vi "ReadInnerValue.vi"(8 "error in (no error)":errorcluster, 11 "Arduino in":refnum<class "Arduino.lvclass">) -> (0 "error out":errorcluster, 3 "Arduino out":refnum<class "Arduino.lvclass">)   [LabVIEW 2013, in "Arduino.lvclass"]
uses:
  Arduino.lvclass
panel:
  out "Value":dbl
  in  "Stop_Marker":string
  in  "Start_Marker":string
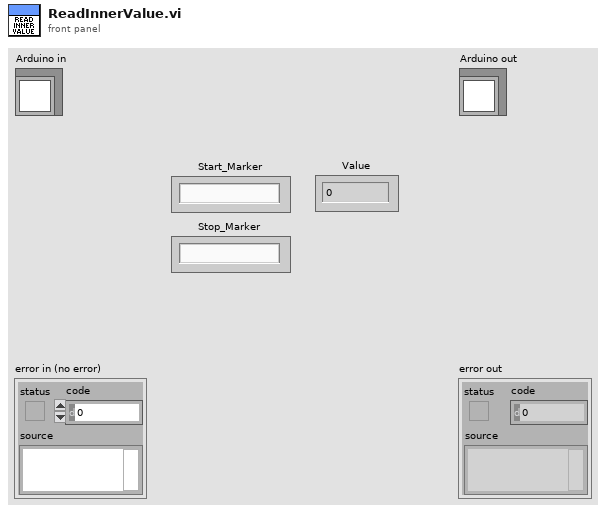
[diagram p1: front panel]
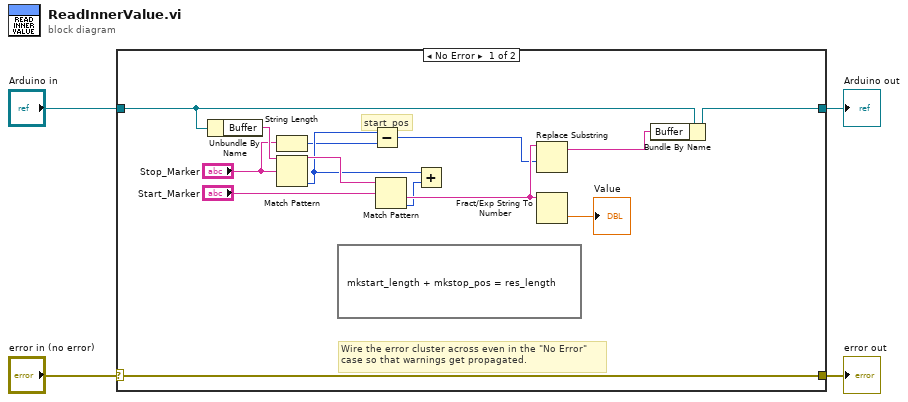
[diagram p0: block diagram]
diagram:
  n1 = case shown="No Error" "error in (no error)" {
    selector: "error in (no error)" -> [w18 w20]
    tunnel: [w18 w20] -> w3
    tunnel: [w12 w19] -> w1
    tunnel: "Arduino in" -> [w13 w19]
    frame No Error {
      # "start_pos"
      # "Wire the error cluster across even in the \"No Error\"\ncase so that warnings get propagated."
      n2 = Unbundle By Name(w13) -> ("Buffer"=w10:string)
      n3 = String Length(string="Stop_Marker") -> (length=w6:i32)
      n4 = Match Pattern(string=w10, regular expression="Stop_Marker") -> (before substring=w17:string, offset past match=w7:i32)  [unwired: 1 in, 2 out]
      n5 = formula code="mkstart_length + mkstop_pos = res_length"() -> ()
      n6 = Subtract(x=w7, y=w6) -> (x-y=w5:i32)
      n7 = Match Pattern(string=w17, regular expression="Start_Marker") -> (after substring=w14:string, offset past match=w8:i32)  [unwired: 1 in, 2 out]
      n8 = Add(x=w7, y=w8) -> ()  [unwired: 1 out]
      n9 = Replace Substring(3:w5, 5:w14) -> (1:w11:string)  [unwired: 2 in, 1 out]
      n10 = Fract/Exp String To Number(string=w14) -> (number=→"Value":dbl)  [unwired: 3 in, 1 out]
      n11 = Bundle By Name(cluster=w13, "Buffer"=w11) -> (w12:refnum<class "Arduino.lvclass">)
    }
    frame Error {
    }
  }
  "error out" <- w3
  "Arduino out" <- w1
